vi "Initialize MeasurementLink Session.vi"(7 "remote connection options":T2, 8 "error in":errorcluster, 9 "initialize session behavior":T1, 10 "session initialization parameters":T3, 11 "session factory in":refnum<class "Session Factory.lvclass">) -> (0 "error out":errorcluster, 2 "session out":variant, 3 "session factory out":refnum<class "Session Factory.lvclass">)   [LabVIEW 2020, in "Keysight 34401A DMM Instrument.lvlib" / "Session Factory.lvclass"]
uses:
  Session Factory.lvclass
  <vilib>/MeasurementLink/MeasurementLink Instrument/ISession Factory/Session Initialization Parameters.ctl
  <vilib>/MeasurementLink/MeasurementLink Instrument/ISession Factory/Remote Connection Options.ctl
  <vilib>/MeasurementLink/MeasurementLink Instrument/ISession Factory/Initialize and Close Session Behavior.ctl
  Session Factory.lvclass/Session Factory.ctl
  <vilib>/MeasurementLink/MeasurementLink Instrument/ISession Factory/ISession Factory.lvclass
  <instrlib>/Agilent 34401/Public/Initialize.vi
  <instrlib>/Agilent 34401/Agilent 34401.lvlib
  <vilib>/NI-VISA/VISA Open for gRPC Session.vi
  Get VISA gRPC Open Close Behavior.vi
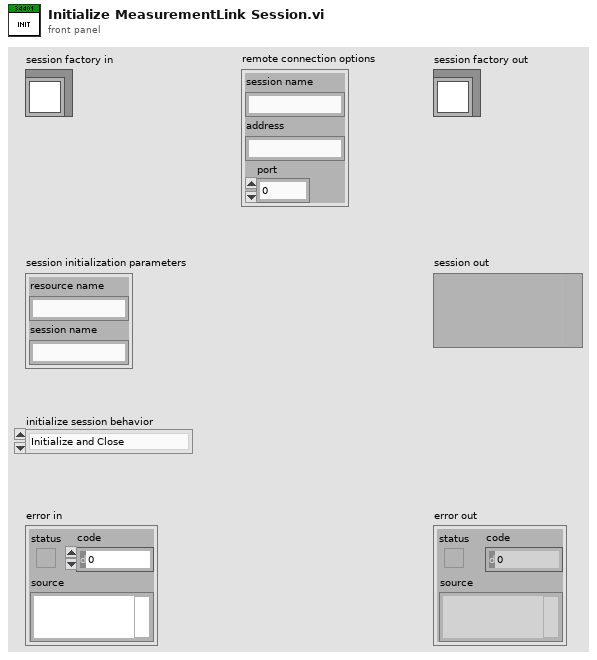
[diagram p1: front panel]
types:
  T1 = typedef "MeasurementLink Instrument.lvlib/ISession Factory.lvclass/Initialize and Close Session Behavior.ctl" = enum16{"Initialize and Close", "Attach and Detach", "Initialize and Detach", "Attach and Close"}
  T2 = typedef "MeasurementLink Instrument.lvlib/ISession Factory.lvclass/Remote Connection Options.ctl" = cluster{"session name":string, "address":string, "port":u32}
  T3 = typedef "MeasurementLink Instrument.lvlib/ISession Factory.lvclass/Session Initialization Parameters.ctl" = cluster{"resource name":string, "session name":string}
  T4 = cluster{"Baud Rate":u32, "Parity":u16, "Data Bits":u16}
  T5 = typedef "VISA gRPC Open Close Behavior.ctl" = enum16{"Auto", "Initialize and Close", "Attach and Detach", "Initialize and Detach", "Attach and Close"}
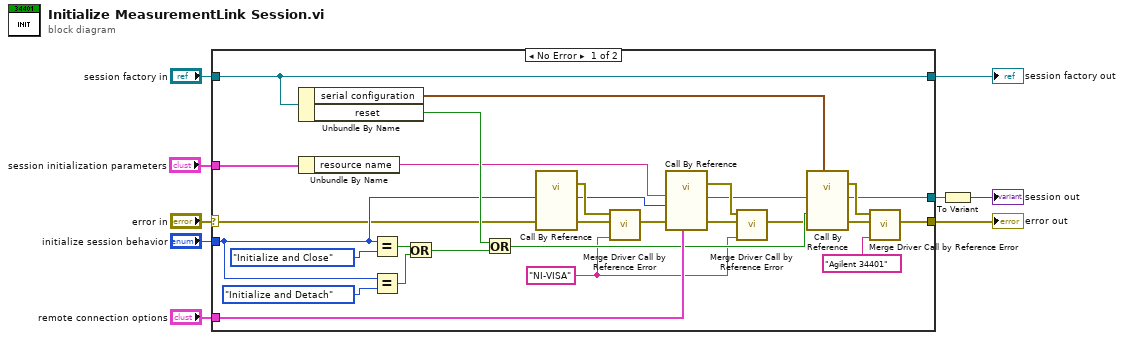
[diagram p0: block diagram]
diagram:
  n1 = case shown="No Error" "error in" {
    selector: "error in" -> [w16 w38]
    tunnel: [w20 w38] -> w8
    tunnel: "session factory in" -> [w36 w39]
    tunnel: [w36 w39] -> w6
    tunnel: "initialize session behavior" -> [w17 _]
    tunnel: "session initialization parameters" -> [w37 _]
    tunnel: "remote connection options" -> [w28 _]
    tunnel: [w19 _] -> w1
    frame No Error {
      w15 = "NI-VISA" ("driver name")
      n2 = Unbundle By Name(w36) -> ("serial configuration"=w10:T4, "reset"=w34:bool)
      n3 = Unbundle By Name(w37) -> ("resource name"=w29:string)
      n4 = Equal?(x=w17, y=Initialize_and_Close_Session_Behavior."Initialize and Close" ("initialize session behavior")) -> (x = y?=w31:bool)
      n5 = Equal?(x=w17, y=Initialize_and_Close_Session_Behavior."Initialize and Detach" ("initialize session behavior")) -> (x = y?=w30:bool)
      n6 = Or(x=w31, y=w30) -> (x .or. y?=w33:bool)
      n7 = Or(x=w34, y=w33) -> (x .or. y?=w27:bool)
      n8 = call-by-ref "?"("error in (no error)"=w16, "initialize session behavior"=w17) -> (error out=w13:errorcluster, 0:"error out"=w14:errorcluster, "open/close behavior"=w11:T5)  [unwired: 10 in, 1 out]
      n9 = call <vilib>:"Merge Driver Call by Reference Error.vi"("driver name"=w15, "called vi error"=w14, "call by ref error"=w13) -> ("error out"=w12:errorcluster)  [unwired: 8 in]
      n10 = call-by-ref "?"("gRPC Options"=w28, "error in (no error)"=w12, "Open/Close Behavior"=w11, "VISA resource name"=w29) -> (error out=w25:errorcluster, 0:"error out"=w24:errorcluster, "VISA resource name out"=w18:refnum<visa-resource-name>)  [unwired: 8 in, 1 out]
      n11 = call <vilib>:"Merge Driver Call by Reference Error.vi"("driver name"=w15, "called vi error"=w24, "call by ref error"=w25) -> ("error out"=w22:errorcluster)  [unwired: 8 in]
      n12 = call-by-ref "?"("Serial Configuration"=w10, "error in (no error)"=w22, "Reset (True)"=w27, "VISA resource name"=w18) -> (error out=w26:errorcluster, 0:"error out"=w21:errorcluster, "VISA resource name out"=w19:refnum<visa-resource-name>)  [unwired: 8 in, 1 out]
      n13 = call <vilib>:"Merge Driver Call by Reference Error.vi"("driver name"="Agilent 34401", "called vi error"=w21, "call by ref error"=w26) -> ("error out"=w20:errorcluster)  [unwired: 8 in]
    }
    frame Error {
    }
  }
  "error out" <- w8
  "session factory out" <- w6
  n14 = To Variant(anything=w1) -> (Variant=→"session out":variant)
